vi "monitor stop notification.vi"(11 "Template in":refnum<class "Template.lvclass">) -> (3 "Stop?":bool)   [LabVIEW 2020, in "Template.lvlib" / "Template.lvclass"]
doc: "Returns True if notification is generated or the Notifier is released from memory.\nUse this to stop loops that are not commanded by an Event structure"
uses:
  Template.lvclass
  Template.lvclass/Template.ctl
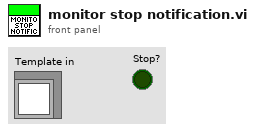
[diagram p1: front panel]
types:
  T1 = typedef "Template.lvlib/Template.lvclass/base actor notifiers.ctl" = cluster{"Stop Actor":refnum<notifier>, "UI Data":refnum<notifier>}
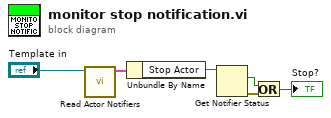
[diagram p0: block diagram]
diagram:
  n1 = call "Read Actor Notifiers.vi"("Template in"="Template in") -> ("Base Actor Notifiers"=w5:T1)  [unwired: 10 in]
  n2 = Unbundle By Name(w5) -> ("Stop Actor"=w4:refnum<notifier>)
  n3 = Get Notifier Status(notifier=w4) -> (current notification=w3:bool, error out=w1:errorcluster)  [unwired: 1 in, 3 out]
  n4 = Or(x=w3, y=w1) -> (x .or. y?=→"Stop?":bool)
